vi "M9300A_status.vi"(8 "error in (no error)":errorcluster {"code" format="%.0x"}, 11 "instrument handle in":refnum<k15>) -> (0 "error out":errorcluster {"code" format="%.0x"}, 2 "Status":bool[](array[boolean]), 3 "instrument handle out":refnum<k15>)   [LabVIEW 2023]
uses:
  Program Files (x86)/Agilent/M938x/LabVIEW Driver/20xx/Agilent M9300/Agilent M9300.lvlib
panel:
  # "ch1 ch2 ch3 ch4  ch5   bp   10m  xo  br    ext"
  # "100MHz channel 1-5\nbp_out\nref_10_MHZ_OUT\nOCXO\nBACK_PLANE_REFERENCE\nEXTERNAL_REFERENCE"
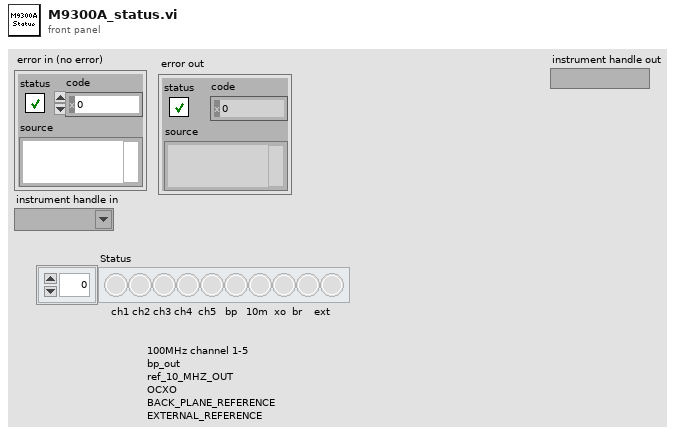
[diagram p1: front panel]
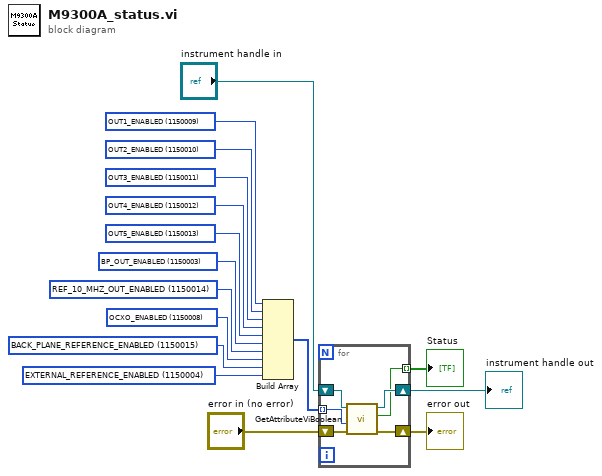
[diagram p0: block diagram]
diagram:
  w3 = u32 1150004 items=["BACK_PLANE_REFERENCE_ENABLED"=1150015, "BP_OUT_ENABLED"=1150003, "EXTERNAL_REFERENCE_ENABLED"=1150004, "EXTERNAL_REFERENCE_PRESENT"=1150006, "LOCKED"=1150007, "NONVOLATILE_ENABLE_INSTRUMENT_CAL_WARNINGS"=1150029, "NONVOLATILE_ENABLE_MODULE_CAL_WARNINGS"=1150028, "NONVOLATILE_ENABLE_PERIODIC_CAL"=1150027, "OCXO_ENABLED"=1150008, "OUT1_ENABLED"=1150009, "OUT2_ENABLED"=1150010, "OUT3_ENABLED"=1150011, "OUT4_ENABLED"=1150012, "OUT5_ENABLED"=1150013, "PROGRAMMABLE_TRIGGER_ENABLED"=1150033, "REF_10_MHZ_OUT_ENABLED"=1150014, "SIMULATE"=1050005, "TRACE_ENABLED"=1150002] ("AttributeID")
  w8 = u32 1150014 items=["BACK_PLANE_REFERENCE_ENABLED"=1150015, "BP_OUT_ENABLED"=1150003, "EXTERNAL_REFERENCE_ENABLED"=1150004, "EXTERNAL_REFERENCE_PRESENT"=1150006, "LOCKED"=1150007, "NONVOLATILE_ENABLE_INSTRUMENT_CAL_WARNINGS"=1150029, "NONVOLATILE_ENABLE_MODULE_CAL_WARNINGS"=1150028, "NONVOLATILE_ENABLE_PERIODIC_CAL"=1150027, "OCXO_ENABLED"=1150008, "OUT1_ENABLED"=1150009, "OUT2_ENABLED"=1150010, "OUT3_ENABLED"=1150011, "OUT4_ENABLED"=1150012, "OUT5_ENABLED"=1150013, "PROGRAMMABLE_TRIGGER_ENABLED"=1150033, "REF_10_MHZ_OUT_ENABLED"=1150014, "SIMULATE"=1050005, "TRACE_ENABLED"=1150002] ("AttributeID")
  w7 = u32 1150008 items=["BACK_PLANE_REFERENCE_ENABLED"=1150015, "BP_OUT_ENABLED"=1150003, "EXTERNAL_REFERENCE_ENABLED"=1150004, "EXTERNAL_REFERENCE_PRESENT"=1150006, "LOCKED"=1150007, "NONVOLATILE_ENABLE_INSTRUMENT_CAL_WARNINGS"=1150029, "NONVOLATILE_ENABLE_MODULE_CAL_WARNINGS"=1150028, "NONVOLATILE_ENABLE_PERIODIC_CAL"=1150027, "OCXO_ENABLED"=1150008, "OUT1_ENABLED"=1150009, "OUT2_ENABLED"=1150010, "OUT3_ENABLED"=1150011, "OUT4_ENABLED"=1150012, "OUT5_ENABLED"=1150013, "PROGRAMMABLE_TRIGGER_ENABLED"=1150033, "REF_10_MHZ_OUT_ENABLED"=1150014, "SIMULATE"=1050005, "TRACE_ENABLED"=1150002] ("AttributeID")
  w6 = u32 1150015 items=["BACK_PLANE_REFERENCE_ENABLED"=1150015, "BP_OUT_ENABLED"=1150003, "EXTERNAL_REFERENCE_ENABLED"=1150004, "EXTERNAL_REFERENCE_PRESENT"=1150006, "LOCKED"=1150007, "NONVOLATILE_ENABLE_INSTRUMENT_CAL_WARNINGS"=1150029, "NONVOLATILE_ENABLE_MODULE_CAL_WARNINGS"=1150028, "NONVOLATILE_ENABLE_PERIODIC_CAL"=1150027, "OCXO_ENABLED"=1150008, "OUT1_ENABLED"=1150009, "OUT2_ENABLED"=1150010, "OUT3_ENABLED"=1150011, "OUT4_ENABLED"=1150012, "OUT5_ENABLED"=1150013, "PROGRAMMABLE_TRIGGER_ENABLED"=1150033, "REF_10_MHZ_OUT_ENABLED"=1150014, "SIMULATE"=1050005, "TRACE_ENABLED"=1150002] ("AttributeID")
  w9 = u32 1150003 items=["BACK_PLANE_REFERENCE_ENABLED"=1150015, "BP_OUT_ENABLED"=1150003, "EXTERNAL_REFERENCE_ENABLED"=1150004, "EXTERNAL_REFERENCE_PRESENT"=1150006, "LOCKED"=1150007, "NONVOLATILE_ENABLE_INSTRUMENT_CAL_WARNINGS"=1150029, "NONVOLATILE_ENABLE_MODULE_CAL_WARNINGS"=1150028, "NONVOLATILE_ENABLE_PERIODIC_CAL"=1150027, "OCXO_ENABLED"=1150008, "OUT1_ENABLED"=1150009, "OUT2_ENABLED"=1150010, "OUT3_ENABLED"=1150011, "OUT4_ENABLED"=1150012, "OUT5_ENABLED"=1150013, "PROGRAMMABLE_TRIGGER_ENABLED"=1150033, "REF_10_MHZ_OUT_ENABLED"=1150014, "SIMULATE"=1050005, "TRACE_ENABLED"=1150002] ("AttributeID")
  w10 = u32 1150013 items=["BACK_PLANE_REFERENCE_ENABLED"=1150015, "BP_OUT_ENABLED"=1150003, "EXTERNAL_REFERENCE_ENABLED"=1150004, "EXTERNAL_REFERENCE_PRESENT"=1150006, "LOCKED"=1150007, "NONVOLATILE_ENABLE_INSTRUMENT_CAL_WARNINGS"=1150029, "NONVOLATILE_ENABLE_MODULE_CAL_WARNINGS"=1150028, "NONVOLATILE_ENABLE_PERIODIC_CAL"=1150027, "OCXO_ENABLED"=1150008, "OUT1_ENABLED"=1150009, "OUT2_ENABLED"=1150010, "OUT3_ENABLED"=1150011, "OUT4_ENABLED"=1150012, "OUT5_ENABLED"=1150013, "PROGRAMMABLE_TRIGGER_ENABLED"=1150033, "REF_10_MHZ_OUT_ENABLED"=1150014, "SIMULATE"=1050005, "TRACE_ENABLED"=1150002] ("AttributeID")
  w11 = u32 1150012 items=["BACK_PLANE_REFERENCE_ENABLED"=1150015, "BP_OUT_ENABLED"=1150003, "EXTERNAL_REFERENCE_ENABLED"=1150004, "EXTERNAL_REFERENCE_PRESENT"=1150006, "LOCKED"=1150007, "NONVOLATILE_ENABLE_INSTRUMENT_CAL_WARNINGS"=1150029, "NONVOLATILE_ENABLE_MODULE_CAL_WARNINGS"=1150028, "NONVOLATILE_ENABLE_PERIODIC_CAL"=1150027, "OCXO_ENABLED"=1150008, "OUT1_ENABLED"=1150009, "OUT2_ENABLED"=1150010, "OUT3_ENABLED"=1150011, "OUT4_ENABLED"=1150012, "OUT5_ENABLED"=1150013, "PROGRAMMABLE_TRIGGER_ENABLED"=1150033, "REF_10_MHZ_OUT_ENABLED"=1150014, "SIMULATE"=1050005, "TRACE_ENABLED"=1150002] ("AttributeID")
  w12 = u32 1150011 items=["BACK_PLANE_REFERENCE_ENABLED"=1150015, "BP_OUT_ENABLED"=1150003, "EXTERNAL_REFERENCE_ENABLED"=1150004, "EXTERNAL_REFERENCE_PRESENT"=1150006, "LOCKED"=1150007, "NONVOLATILE_ENABLE_INSTRUMENT_CAL_WARNINGS"=1150029, "NONVOLATILE_ENABLE_MODULE_CAL_WARNINGS"=1150028, "NONVOLATILE_ENABLE_PERIODIC_CAL"=1150027, "OCXO_ENABLED"=1150008, "OUT1_ENABLED"=1150009, "OUT2_ENABLED"=1150010, "OUT3_ENABLED"=1150011, "OUT4_ENABLED"=1150012, "OUT5_ENABLED"=1150013, "PROGRAMMABLE_TRIGGER_ENABLED"=1150033, "REF_10_MHZ_OUT_ENABLED"=1150014, "SIMULATE"=1050005, "TRACE_ENABLED"=1150002] ("AttributeID")
  w13 = u32 1150010 items=["BACK_PLANE_REFERENCE_ENABLED"=1150015, "BP_OUT_ENABLED"=1150003, "EXTERNAL_REFERENCE_ENABLED"=1150004, "EXTERNAL_REFERENCE_PRESENT"=1150006, "LOCKED"=1150007, "NONVOLATILE_ENABLE_INSTRUMENT_CAL_WARNINGS"=1150029, "NONVOLATILE_ENABLE_MODULE_CAL_WARNINGS"=1150028, "NONVOLATILE_ENABLE_PERIODIC_CAL"=1150027, "OCXO_ENABLED"=1150008, "OUT1_ENABLED"=1150009, "OUT2_ENABLED"=1150010, "OUT3_ENABLED"=1150011, "OUT4_ENABLED"=1150012, "OUT5_ENABLED"=1150013, "PROGRAMMABLE_TRIGGER_ENABLED"=1150033, "REF_10_MHZ_OUT_ENABLED"=1150014, "SIMULATE"=1050005, "TRACE_ENABLED"=1150002] ("AttributeID")
  w14 = u32 1150009 items=["BACK_PLANE_REFERENCE_ENABLED"=1150015, "BP_OUT_ENABLED"=1150003, "EXTERNAL_REFERENCE_ENABLED"=1150004, "EXTERNAL_REFERENCE_PRESENT"=1150006, "LOCKED"=1150007, "NONVOLATILE_ENABLE_INSTRUMENT_CAL_WARNINGS"=1150029, "NONVOLATILE_ENABLE_MODULE_CAL_WARNINGS"=1150028, "NONVOLATILE_ENABLE_PERIODIC_CAL"=1150027, "OCXO_ENABLED"=1150008, "OUT1_ENABLED"=1150009, "OUT2_ENABLED"=1150010, "OUT3_ENABLED"=1150011, "OUT4_ENABLED"=1150012, "OUT5_ENABLED"=1150013, "PROGRAMMABLE_TRIGGER_ENABLED"=1150033, "REF_10_MHZ_OUT_ENABLED"=1150014, "SIMULATE"=1050005, "TRACE_ENABLED"=1150002] ("AttributeID")
  n1 = Build Array(w14, w13, w12, w11, w10, w9, w8, w7, w6, w3) -> (w5:u32[])
  n2 = for {
    shift-right: [w19] -> w1
    shift-left: "instrument handle in" -> [w22]
    shift-right: [w20] -> w15
    shift-left: "error in (no error)" -> [w21]
    tunnel: w5 -> [w18] mode=indexing
    tunnel: [w17] -> w4 mode=indexing
    n3 = call "GetAttributeViBoolean.vi"("error in (no error)"=w21, "AttributeID"=w18, "instrument handle"=w22) -> ("error out"=w20:errorcluster, "AttributeValue"=w17:bool, "instrument handle out"=w19:refnum<k15>)  [unwired: 6 in]
  }
  "error out" <- w15
  "Status" <- w4
  "instrument handle out" <- w1
